vi "Decrypt String.vi"(9 "Crypto Key":string="\u00124Vx\t", 11 "Encrypted String":string) -> (1 "Success":bool, 3 "Decrypted String":string)   [LabVIEW 2018, in "BlowFish.lvlib"]
uses:
  BlowFish.lvlib
panel:
  # "INPUTS"
  # "OUTPUTS"
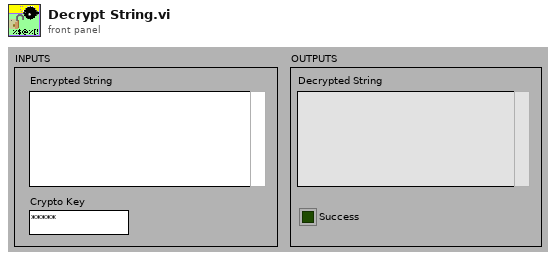
[diagram p1: front panel]
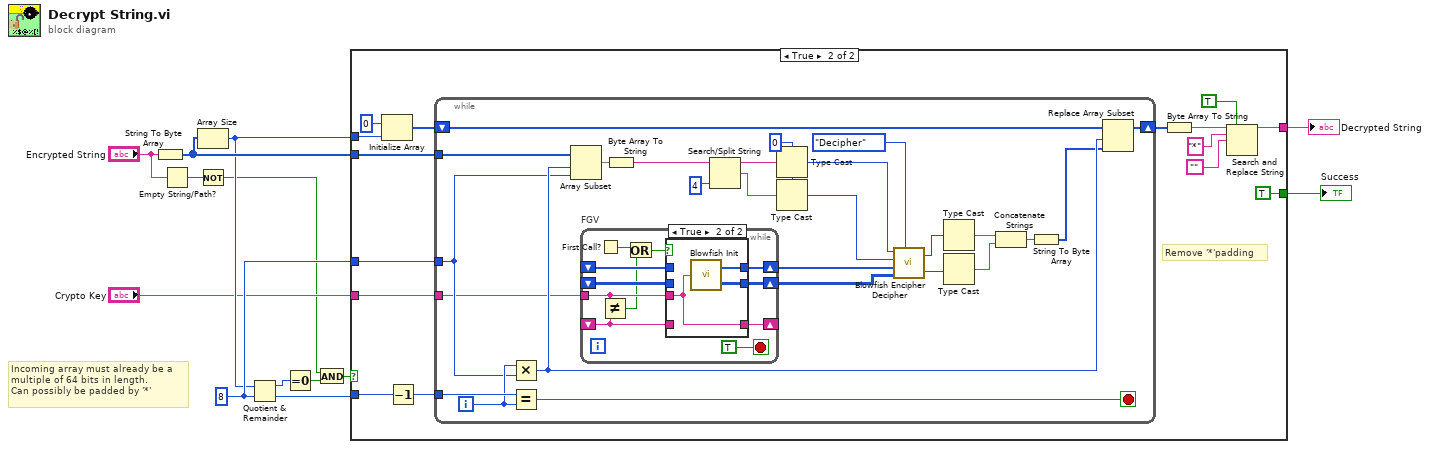
[diagram p0: block diagram]
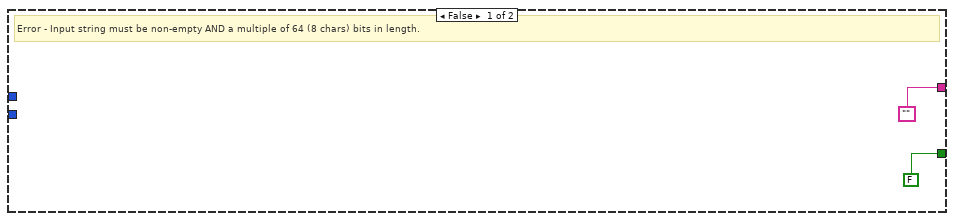
[diagram p2: hidden frame]
diagram:
  w11 = 8 ("y")
  # "Incoming array must already be a\nmultiple of 64 bits in length.\nCan possibly be padded by '*'"
  n1 = String To Byte Array(string="Encrypted String") -> (unsigned byte array=w12:u8[])
  n2 = Empty String/Path?(string/path="Encrypted String") -> (empty?=w5:bool)
  n3 = Array Size(array=w12) -> (size(s)=w10:i32)
  n4 = Not(x=w5) -> (.not. x?=w2:bool)
  n5 = Quotient & Remainder(x=w10, y=w11) -> (x-y*floor(x/y)=w9:i32, floor(x/y)=w13:i32)
  n6 = Equal To 0?(x=w9) -> (x = 0?=w4:bool)
  n7 = And(x=w2, y=w4) -> (x .and. y?=w3:bool)
  n8 = case shown="True" w3 {
    tunnel: w13 -> [_ w27]
    tunnel: w12 -> [_ w25]
    tunnel: w11 -> [_ w24]
    tunnel: w10 -> [_ w20]
    tunnel: "Crypto Key" -> [_ w19]
    tunnel: ["" w17] -> w7
    tunnel: [FALSE ("Success") TRUE ("Success")] -> w1
    frame False {
      # "Error - Input string must be non-empty AND a multiple of 64 (8 chars) bits in length."
    }
    frame True {
      # "Remove '*'padding"
      n9 = Initialize Array(u8 0 ("element"), w20) -> (w29:u8[])
      n10 = Decrement(x=w27) -> (x-1=w26:i32)
      n11 = while {
        tunnel: w25 -> [w46]
        tunnel: w26 -> [w37]
        tunnel: w24 -> [w34]
        shift-right: [w38] -> w28
        shift-left: w29 -> [w40]
        tunnel: w19 -> [w33]
        i -> [w35]
        stop <- w36 stop-if-true
        w49 = u32 0
        n12 = Multiply(x=w35, y=w34) -> (x*y=w41:i32)
        n13 = Equal?(x=w37, y=w35) -> (x = y?=w36:bool)
        n14 = Array Subset(array=w46, index=w41, length=w34) -> (w45:u8[])
        n15 = while "FGV" {
          tunnel: w33 -> [w59]
          shift-right: [w67] -> w32
          shift-left: _ -> [w63]
          shift-right: [w66] -> w31
          shift-left: _ -> [w62]
          shift-right: [w61] -> _
          shift-left: _ -> [w58]
          stop <- TRUE stop-if-true
          n16 = First Call?() -> (First Call?: T/F=w64:bool)
          n17 = Not Equal?(x=w59, y=w58) -> (x != y?=w57:bool)
          n18 = Or(x=w64, y=w57) -> (x .or. y?=w60:bool)
          n19 = case shown="True" w60 {
            tunnel: [w70 w73] -> w67
            tunnel: [w69 w72] -> w66
            tunnel: w59 -> [_ w71]
            tunnel: w63 -> [w70 _]
            tunnel: w62 -> [w69 _]
            tunnel: [w68 w71] -> w61
            tunnel: w58 -> [w68 _]
            frame False {
            }
            frame True {
              n20 = call "Blowfish Init.vi"("Key"=w71) -> ("P 18"=w73:u32[], "S 4X256"=w72:u32[][])
            }
          }
        }
        n21 = Byte Array To String(unsigned byte array=w45) -> (string=w44:string)
        n22 = Search/Split String(string=w44, offset (0)=4) -> (substring before match=w55:string, match + rest of string=w56:string)  [unwired: 1 in, 1 out]
        n23 = Type Cast(type=w49, x=w55) -> (*(type *) &x=w48:u32)
        n24 = Type Cast(type=w49, x=w56) -> (*(type *) &x=w47:u32)
        n25 = call "Blowfish Encipher Decipher.vi"("Xl"=w48, "Xr"=w47, "P 18"=w32, "S 4X256"=w31, "Enc/Dec"=enum16{"Encipher", "Decipher"}."Decipher") -> ("Xl out"=w50:u32, "Xr out"=w51:u32)
        n26 = Type Cast(x=w50) -> (*(type *) &x=w52:string)  [unwired: 1 in]
        n27 = Type Cast(x=w51) -> (*(type *) &x=w53:string)  [unwired: 1 in]
        n28 = Concatenate Strings(w52, w53) -> (w42:string)
        n29 = String To Byte Array(string=w42) -> (unsigned byte array=w39:u8[])
        n30 = Replace Array Subset(array=w40, new element=w39, index=w41) -> (w38:u8[])
      }
      n31 = Byte Array To String(unsigned byte array=w28) -> (string=w23:string)
      n32 = Search and Replace String(replace all?=TRUE ("replace all? (F)"), input string=w23, search string="*", replace string="") -> (result string=w17:string)  [unwired: 4 in, 3 out]
    }
  }
  "Decrypted String" <- w7
  "Success" <- w1
